vi "Host - Watchdog Close (SubVI).vi"(8 "error in":errorcluster) -> (0 "error out":errorcluster)   [LabVIEW 2021]
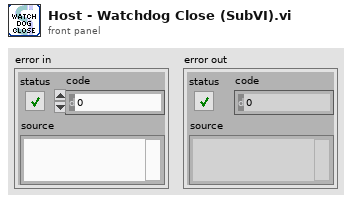
[diagram p1: front panel]
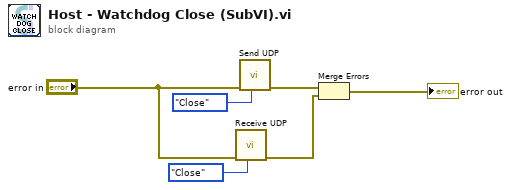
[diagram p0: block diagram]
diagram:
  n1 = call "Receive UDP.vi"("Operation"=enum16{"Init", "Receive", "Close"}."Close", "error in"="error in") -> ("error out"=w1:errorcluster)  [unwired: 7 in, 2 out]
  n2 = call "Send UDP.vi"("Operation"=enum16{"Init", "Send", "Close"}."Close", "error in"="error in") -> ("error out"=w2:errorcluster)  [unwired: 8 in, 1 out]
  n3 = Merge Errors(w2, w1) -> (→"error out":errorcluster)
